vi "Construct Control Event.vi"(9 "GObject in":refnum<vi>, 10 "Event Type":T1) -> (2 "Event":T2)   [LabVIEW 2015, in "Scripting.lvlib"]
doc: "Contructs a set of events for single event frame that contains only a single Static Control Event."
uses:
  Scripting.lvlib
  <vilib>/event_ctls.llb/lveventtype.ctl
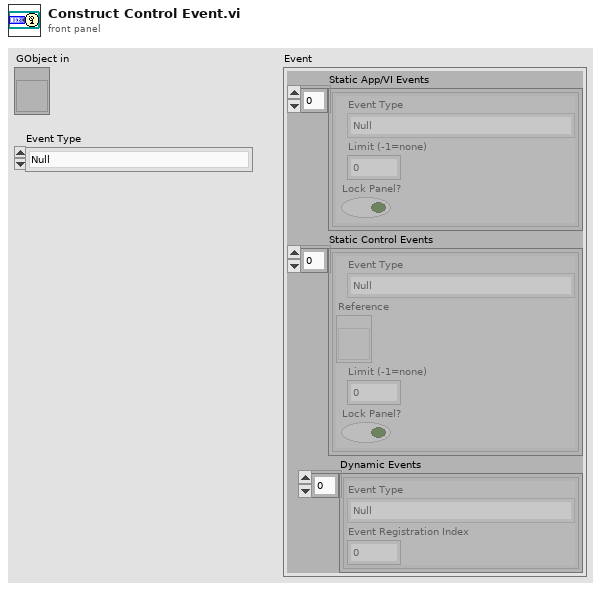
[diagram p1: front panel]
types:
  T1 = typedef "lveventtype.ctl" = enum32{"Null", "Timeout", "Annotation Menu Selection", "Annotation Menu Selection?", "App Instance Close", "App Instance Close?", "Autoscale Range Change", "Bookmark Info Change", "Cell Edit", "Cell Edit?", "Cursor Grab", "Cursor Grab?", "Cursor Menu Selection", "Cursor Menu Selection?", "Cursor Move", "Cursor Release", "Data Change", "Direction Change", "Display State Change", "Drag Ended", "Drag Enter", "Drag Leave", "Drag Over", "Drag Source Update", "Drag Starting", "Drag Starting?", "Drop", "Exec State Change", "Key Down", "Key Down?", "Key Repeat", "Key Repeat?", "Key Up", "Listbox Double Click", "Menu Activation?", "Menu Selection (App)", "Menu Selection? (App)", "Menu Selection (User)", "Mouse Down", "Mouse Down?", "Mouse Enter", "Mouse Leave", "Mouse Move", "Mouse Up", "Mouse Wheel", "NI Security User Change (App)", "Pane Size", "Panel Close", "Panel Close?", "Panel Resize", "Plot Attribute Change", "Scale Range Change", "Shortcut Menu Activation?", "Shortcut Menu Selection (App)", "Shortcut Menu Selection? (App)", "Shortcut Menu Selection (User)", "Tree Double Click", "Tree Drag", "Tree Drag?", "Tree Drop", "Tree Drop?", "Tree Item Close", "Tree Item Close?", "Tree Item Open", "Tree Item Open?", "User Event", "Value Change"}
  T2 = cluster{"Static App/VI Events":cluster{"Event Type":T1, "Limit (-1=none)":i32, "Lock Panel?":bool}[], "Static Control Events":cluster{"Event Type":T1, "Reference":refnum<vi>, "Limit (-1=none)":i32, "Lock Panel?":bool}[], "Dynamic Events":cluster{"Event Type":T1, "Event Registration Index":i32}[]}
  T3 = cluster{"Event Type":T1, "Reference":refnum<vi>, "Limit (-1=none)":i32, "Lock Panel?":bool}
  T4 = cluster{"Event Type":T1, "Reference":refnum<vi>, "Limit (-1=none)":i32, "Lock Panel?":bool}[]
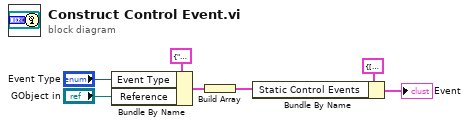
[diagram p0: block diagram]
diagram:
  n1 = Bundle By Name(cluster=T3 {"Event Type"=enum."Value Change", "Reference"=refnum, "Limit (-1=none)"=-1, "Lock Panel?"=FALSE} ("Static Control Events"), "Event Type"="Event Type", "Reference"="GObject in") -> (w3:T3)
  n2 = Build Array(w3) -> (w4:T4)
  n3 = Bundle By Name(cluster=T2 {"Static App/VI Events"=[], "Static Control Events"=[], "Dynamic Events"=[]}, "Static Control Events"=w4) -> (→"Event":T2)
